vi "Remove.vi"(8 "error in (no error)":errorcluster caption="错误输入（无错误）", 10 "Key":variant, 11 "HashTable 输入":refnum<class "HashTable.lvclass"> caption="DNL_LabVIEW Object in") -> (0 "error out":errorcluster caption="错误输出", 3 "HashTable 输出":refnum<class "HashTable.lvclass"> caption="DNL_LabVIEW Object out")   [LabVIEW 2012, in "HashTable.lvclass"]
uses:
  HashTable.lvclass
  HashTable.lvclass/HashTable.ctl
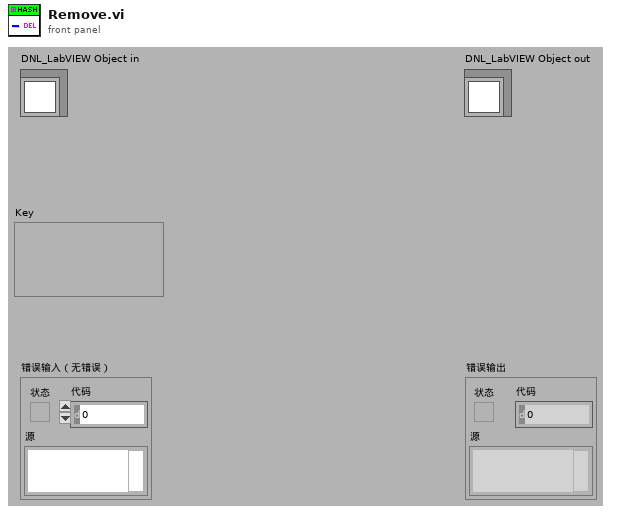
[diagram p1: front panel]
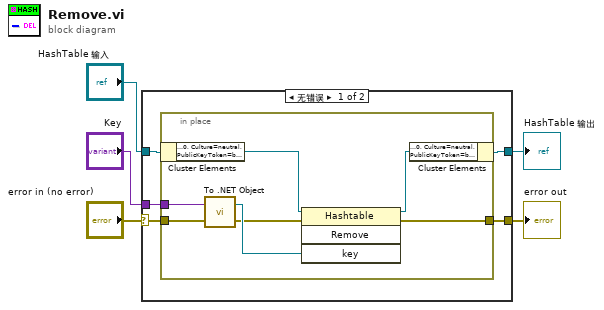
[diagram p0: block diagram]
diagram:
  n1 = case shown="无错误" "error in (no error)" {
    selector: "error in (no error)" -> [w7 w19]
    tunnel: [w6 w19] -> w4
    tunnel: [w9 w18] -> w2
    tunnel: "HashTable 输入" -> [w10 w18]
    tunnel: "Key" -> [w8 _]
    frame No Error {
      n2 = in-place {
        in-place-border: w8 -> [w14]
        in-place-border: w7 -> [w13]
        in-place-border: [w11] -> w6
        n3 = in-place-cluster #1(w10) -> ("HashTable"=w17:refnum<k24>)
        n4 = call <vilib>:"To .NET Object.vi"("error in (no error)"=w13, "anything"=w14) -> ("error out"=w12:errorcluster, ".NET object"=w15:refnum<k24>)
        n5 = invoke class="Hashtable" method="Remove"(reference=w17, error in=w12, "key"=w15) -> (reference out=w16:refnum<k24>, error out=w11:errorcluster)  [unwired: 1 in, 2 out]
        n6 = in-place-cluster #1("HashTable"=w16) -> (w9:refnum<class "HashTable.lvclass">)
      }
    }
    frame Error {
    }
  }
  "error out" <- w4
  "HashTable 输出" <- w2
